vi "RFScan.vi"() -> ()   [LabVIEW 2014]
panel:
  in  "Parameter":u16(ring) items=["Frequency (MHz)", "Amplitude (dBm)"]
  in  "Start":dbl=1.0 format="%.4f"
  in  "End":dbl=10.0 format="%.4f"
  in  "Step":dbl=0.1 format="%.4f"
  in  "RF Scan":bool
  in  "Frequency (MHz)":dbl=1000.0 format="%.4f"
  in  "Amplitude (dBm)":dbl=-40.0 format="%.2f"
  in  "Device":u32(ring) items=["Cooling", "13G", "1G"]
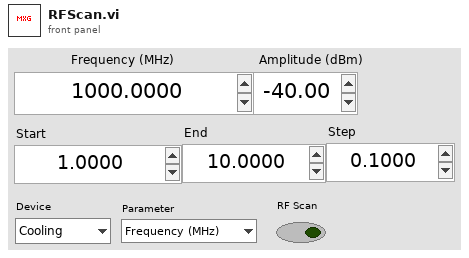
[diagram p1: front panel]
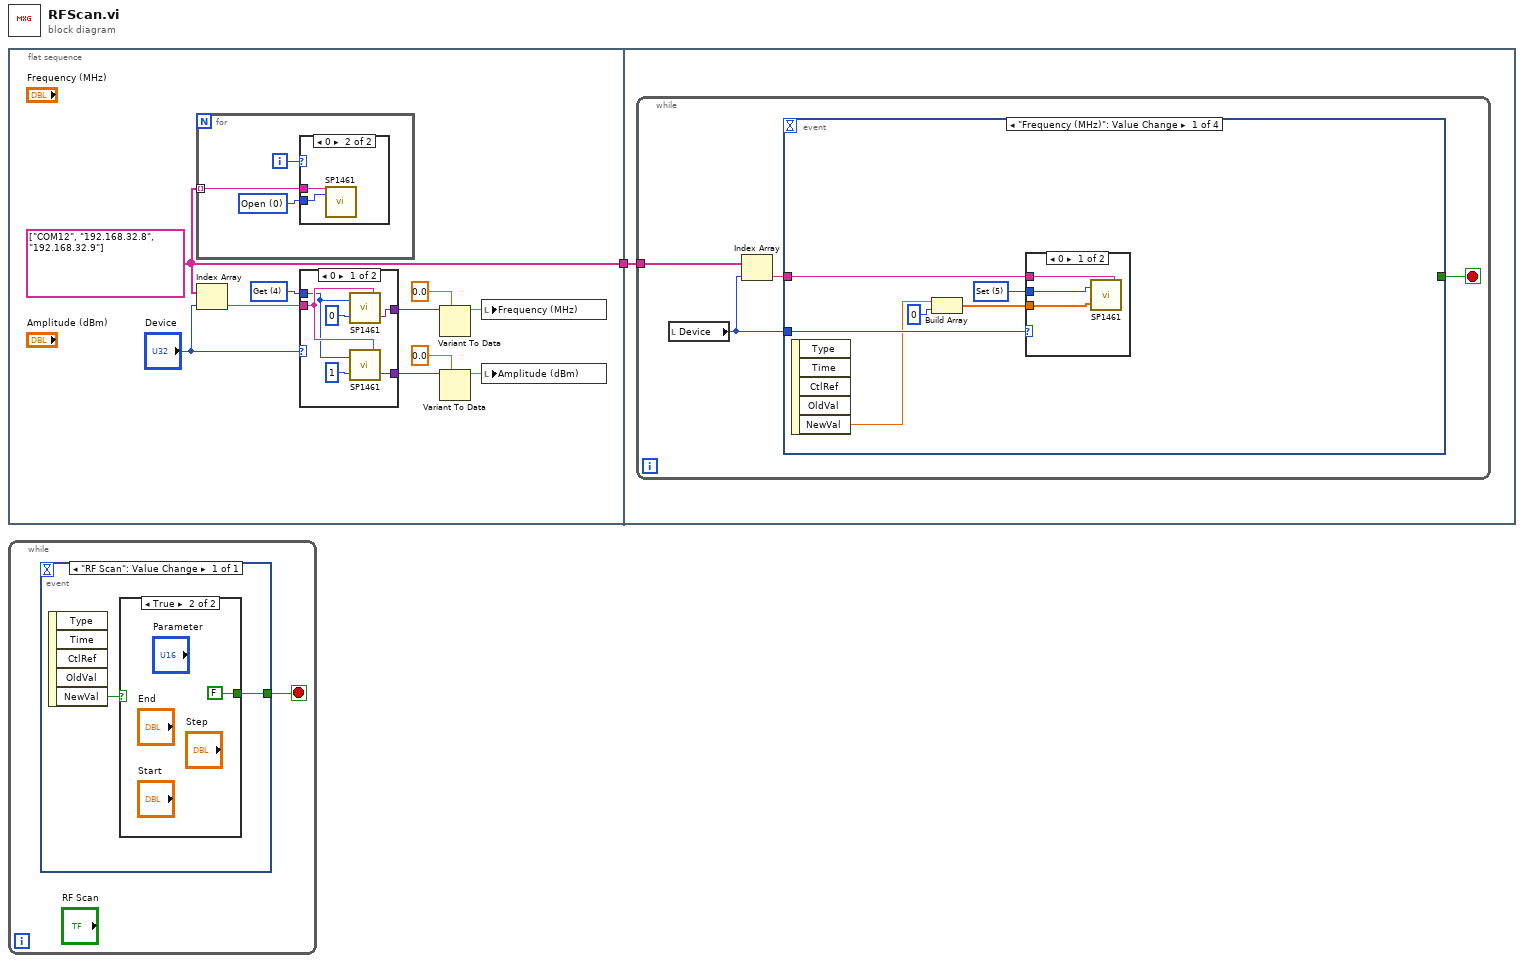
[diagram p0: block diagram]
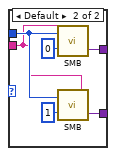
[diagram p3: hidden frame]
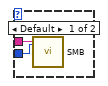
[diagram p4: hidden frame]
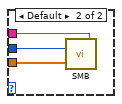
[diagram p5: hidden frame]
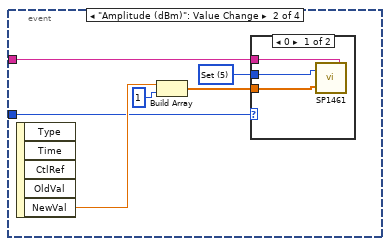
[diagram p6: hidden frame]
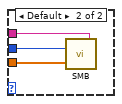
[diagram p7: hidden frame]
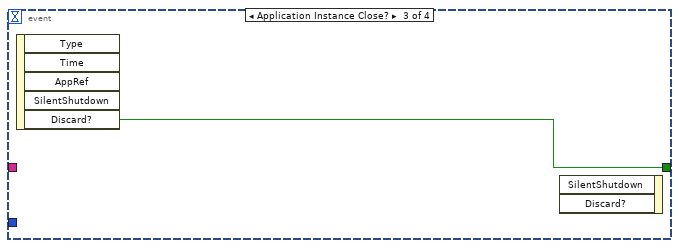
[diagram p8: hidden frame]
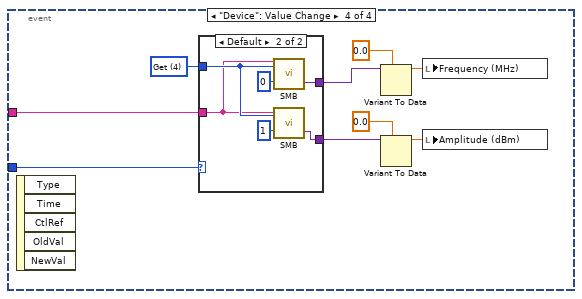
[diagram p9: hidden frame]
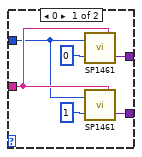
[diagram p10: hidden frame]
diagram:
  n1 = flat-sequence {
    tunnel: [w2] -> w1
    tunnel: w1 -> [w31]
    frame #0 {
      w11 = u32 4 items=["Open", "Close", "Begin", "End", "Get", "Set"] ("Mode")
      w2 = string[] ["COM12", "192.168.32.8", "192.168.32.9"] ("array of strings")
      n2 = for {
        tunnel: w2 -> [w26] mode=indexing
        i -> [w25]
        w24 = u32 0 items=["Open", "Close", "Begin", "End", "Get", "Set"] ("Mode")
        n3 = case shown="0" w25 {
          tunnel: w24 -> [w28 w30]
          tunnel: w26 -> [w27 w29]
          frame Default {
            n4 = call "SMB.vi"("IP"=w27, "Mode"=w28) -> ()  [unwired: 1 in, 1 out]
          }
          frame 0 {
            n5 = call "SP1461.vi"("Port"=w29, "Mode"=w30) -> ()  [unwired: 1 in, 1 out]
          }
        }
      }
      n6 = Index Array(array=w2, index="Device") -> (element=w9:string)
      n7 = case shown="0" "Device" {
        tunnel: w11 -> [w14 w21]
        tunnel: w9 -> [w15 w20]
        tunnel: [w13 w19] -> w4
        tunnel: [w12 w18] -> w3
        frame 0 {
          n8 = call "SP1461.vi"("Port"=w15, "In"=0, "Mode"=w14) -> ("Out"=w13:variant)
          n9 = call "SP1461.vi"("Port"=w15, "In"=1, "Mode"=w14) -> ("Out"=w12:variant)
        }
        frame Default {
          n10 = call "SMB.vi"("IP"=w20, "In"=0, "Mode"=w21) -> ("Out"=w19:variant)
          n11 = call "SMB.vi"("IP"=w20, "In"=1, "Mode"=w21) -> ("Out"=w18:variant)
        }
      }
      n12 = Variant To Data(type=0.0 ("Frequency (MHz)"), Variant=w4) -> (data=w6:dbl)  [unwired: 1 in, 1 out]
      n13 = Variant To Data(type=0.0 ("Frequency (MHz)"), Variant=w3) -> (data=w5:dbl)  [unwired: 1 in, 1 out]
      n14 = local write "Frequency (MHz)"(w6) -> ()
      n15 = local write "Amplitude (dBm)"(w5) -> ()
    }
    frame #1 {
      n16 = while {
        tunnel: w31 -> [w34]
        stop <- w35 stop-if-true
        n17 = local read "Device"() -> (w32:u32)
        n18 = Index Array(array=w34, index=w32) -> (element=w33:string)
        n19 = event shown="[0] \"Frequency (MHz)\": Value Change" {
          selector: _ -> [_ _ _ _]
          dyn-events: _ -> [_ _ _ _]
          timeout: _ -> [_ _ _ _]
          tunnel: [_ _ w60 _] -> w35
          tunnel: w33 -> [w40 w49 _ w62]
          tunnel: w32 -> [w39 w48 _ w61]
          event "Frequency (MHz)": Value Change {
            w41 = u32 5 items=["Open", "Close", "Begin", "End", "Get", "Set"] ("Mode")
            n20 = event-data() -> ("NewVal"=w38:dbl)  [unwired: 1 in, 4 out]
            n21 = Build Array(w38, 0) -> (w36:dbl[])
            n22 = case shown="0" w39 {
              tunnel: w41 -> [w43 w47]
              tunnel: w40 -> [w44 w46]
              tunnel: w36 -> [w42 w45]
              frame 0 {
                n23 = call "SP1461.vi"("Port"=w44, "In"=w42, "Mode"=w43) -> ()  [unwired: 1 out]
              }
              frame Default {
                n24 = call "SMB.vi"("IP"=w46, "In"=w45, "Mode"=w47) -> ()  [unwired: 1 out]
              }
            }
          }
          event "Amplitude (dBm)": Value Change {
            w53 = u32 5 items=["Open", "Close", "Begin", "End", "Get", "Set"] ("Mode")
            n25 = event-data() -> ("NewVal"=w50:dbl)  [unwired: 1 in, 4 out]
            n26 = Build Array(w50, 1) -> (w51:dbl[])
            n27 = case shown="0" w48 {
              tunnel: w53 -> [w55 w59]
              tunnel: w49 -> [w56 w58]
              tunnel: w51 -> [w54 w57]
              frame 0 {
                n28 = call "SP1461.vi"("Port"=w56, "In"=w54, "Mode"=w55) -> ()  [unwired: 1 out]
              }
              frame Default {
                n29 = call "SMB.vi"("IP"=w58, "In"=w57, "Mode"=w59) -> ()  [unwired: 1 out]
              }
            }
          }
          event Application Instance Close? {
            n30 = event-data() -> ("Discard?"=w60:bool)  [unwired: 1 in, 4 out]
            n31 = event-data() -> ()  [unwired: 3 in, 1 out]
          }
          event "Device": Value Change {
            w63 = u32 4 items=["Open", "Close", "Begin", "End", "Get", "Set"] ("Mode")
            n32 = event-data() -> ()  [unwired: 1 in, 5 out]
            n33 = case shown="Default" w61 {
              tunnel: w63 -> [w72 w79]
              tunnel: w62 -> [w73 w78]
              tunnel: [w71 w77] -> w68
              tunnel: [w70 w76] -> w69
              frame 0 {
                n34 = call "SP1461.vi"("Port"=w73, "In"=0, "Mode"=w72) -> ("Out"=w71:variant)
                n35 = call "SP1461.vi"("Port"=w73, "In"=1, "Mode"=w72) -> ("Out"=w70:variant)
              }
              frame Default {
                n36 = call "SMB.vi"("IP"=w78, "In"=0, "Mode"=w79) -> ("Out"=w77:variant)
                n37 = call "SMB.vi"("IP"=w78, "In"=1, "Mode"=w79) -> ("Out"=w76:variant)
              }
            }
            n38 = Variant To Data(type=0.0 ("Frequency (MHz)"), Variant=w68) -> (data=w66:dbl)  [unwired: 1 in, 1 out]
            n39 = Variant To Data(type=0.0 ("Frequency (MHz)"), Variant=w69) -> (data=w67:dbl)  [unwired: 1 in, 1 out]
            n40 = local write "Frequency (MHz)"(w66) -> ()
            n41 = local write "Amplitude (dBm)"(w67) -> ()
          }
        }
      }
    }
  }
  n42 = while {
    stop <- w82 stop-if-true
    n43 = event shown="[0] \"RF Scan\": Value Change" {
      selector: _ -> [_]
      dyn-events: _ -> [_]
      timeout: _ -> [_]
      tunnel: [w84] -> w82
      event "RF Scan": Value Change {
        n44 = event-data() -> ("NewVal"=w83:bool)  [unwired: 1 in, 4 out]
        n45 = case shown="True" w83 {
          tunnel: [_ FALSE ("AWG Scan")] -> w84
          frame False {
          }
          frame True {
          }
        }
      }
    }
  }
